vi "Untitled 7 (SubVI).vi"(8 "error in (no error)":errorcluster, 10 "Angle for pattern (degrees)":sgl, 11 "Refnum in":T3) -> (0 "error out":errorcluster, 1 "Number of Matches (Geometric Matching 1)":i32, 2 "Image Out":T2, 3 "Refnum out":T3, 4 "Calibrated Matches (Geometric Matching 1)":T1[](array[typedef]) {"Correlation Score" format="%.2f"; "Target Template Curve Score" format="%.2f"; "Template Target Curve Score" format="%.2f"; "Bounding Box"."y" format="%.2f"; "Bounding Box"."x" format="%.2f"; "Position"."y" format="%.2f"; "Position"."x" format="%.2f"; "Score" format="%.2f"; "Scale" format="%.2f"; "Angle" format="%.2f"; "Occlusion %" format="%.2f"}, 5 "Image Dst Out":T2)   [LabVIEW 2017]
uses:
  <vilib>/userdefined/High Color/IMAQdx.ctl
  <vilib>/vision/Image Controls.llb/IMAQ Image.ctl
  <vilib>/vision/Pattern Matching.llb/IMAQ GM Match Report.ctl
  <vilib>/vision/NI_Vision_Development_Module.lvlib
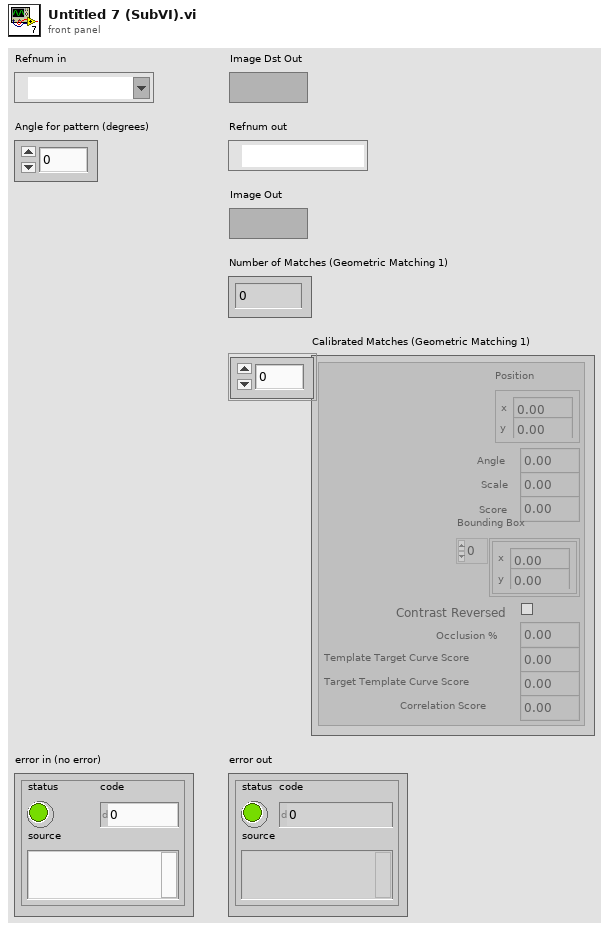
[diagram p1: front panel]
types:
  T1 = typedef "IMAQ GM Match Report.ctl" = cluster{"Position":cluster{"x":sgl, "y":sgl}, "Angle":sgl, "Scale":sgl, "Score":sgl, "Bounding Box":cluster{"x":sgl, "y":sgl}[], "Contrast Reversed":bool, "Occlusion %":sgl, "Template Target Curve Score":sgl, "Target Template Curve Score":sgl, "Correlation Score":sgl}
  T2 = typedef "IMAQ Image.ctl" = refnum<image>
  T3 = typedef "IMAQdx.ctl" = refnum<k21>
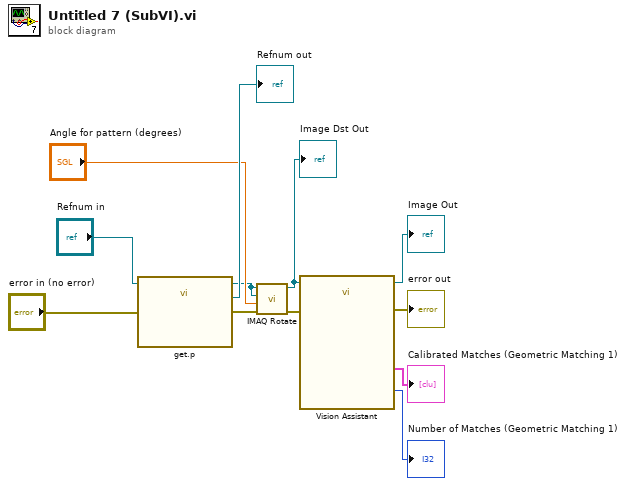
[diagram p0: block diagram]
diagram:
  n1 = call "get.p.vi"("Session in"="Refnum in", "error in"="error in (no error)") -> ("Image Out"=w7:T2, "Session Out"=→"Refnum out":T3, "error out"=w9:errorcluster)  [unwired: 23 in]
  n2 = call "IMAQ Rotate"("error in (no error)"=w9, "Angle (degrees)"="Angle for pattern (degrees)", "Image Dst"=w7, "Image Src"=w7) -> ("error out"=w5:errorcluster, "Image Dst Out"=w6:T2)  [unwired: 6 in]
  "Image Dst Out" <- w6
  n3 = call "Vision Assistant"("Image In"=w6, "error in"=w5) -> ("Image Out"=→"Image Out":T2, "Calibrated Matches (Geometric Matching 1)"=→"Calibrated Matches (Geometric Matching 1)":T1[], "Number of Matches (Geometric Matching 1)"=→"Number of Matches (Geometric Matching 1)":i32, "error out"=→"error out":errorcluster)  [unwired: 22 in]
